vi "DeviceOff.vi"(8 "error in (no error)":errorcluster, 11 "ChromaPowerSupplyModel in":refnum<class "ChromaPowerSupplyModel.lvclass">) -> (0 "error out":errorcluster, 3 "ChromaPowerSupplyModel out":refnum<class "ChromaPowerSupplyModel.lvclass">)   [LabVIEW 2018, in "AcPwrPlugins.lvlib" / "ChromaPowerSupplyModel.lvclass"]
doc: "This VI disables the instruments output form either generating or receiving a signal."
uses:
  ChromaPowerSupplyModel.lvclass
  AcPwrBaseClass/AcPwrBase.lvclass
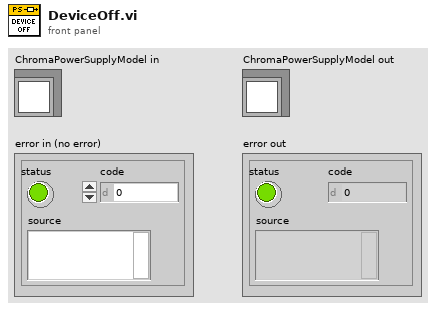
[diagram p1: front panel]
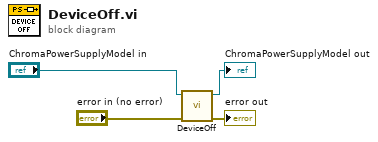
[diagram p0: block diagram]
diagram:
  n1 = call-parent "DeviceOff.vi"("error in (no error)"="error in (no error)", "AcPwrBase in"="ChromaPowerSupplyModel in") -> ("error out"=→"error out":errorcluster, "AcPwrBase out"=→"ChromaPowerSupplyModel out":refnum<class "ChromaPowerSupplyModel.lvclass">)  [unwired: 8 in]
